vi "XVA-DSE7_defaut.vi"(8 "err in":errorcluster, 10 "tmax":dbl, 11 "Weibull (paramètres)":T1) -> (0 "err out":errorcluster, 2 "Graphe Weibull f et R":cluster{dbl[], dbl[]}[](graph) caption="Densité de Probabilité f et Fonction de Répartition F", 3 "X-VA (s)":T2)   [LabVIEW 2010, in "lv_04.lvlib"]
uses:
  lv_04.lvlib
  commandes/cX.ctl
  commandes/cSTA_varid.ctl
  commandes/c_TDMS_ch_variable.ctl
  commandes/c_TDMS_ch_donnees.ctl
  commandes/c0-var-n.ctl
  commandes/cSTA_num_do_cr.ctl
  commandes/c02-do-num.ctl
  commandes/c04-stat-num.ctl
  commandes/cSTA_txt_do_cr.ctl
  commandes/c02-do-txt.ctl
  commandes/c04-stat-txt.ctl
  commandes/cSTA_dist.ctl
  commandes/c03-dist-S.ctl
  commandes/c0-dist-xy.ctl
  commandes/c03-dist-T.ctl
  commandes/c03-dist-SPC.ctl
  lv_02/p_5E7_LW.ctl
  XVA-DSE7-dist.vi
  lv_02/lv_02.lvlib
panel:
  # "Loi Weibull"
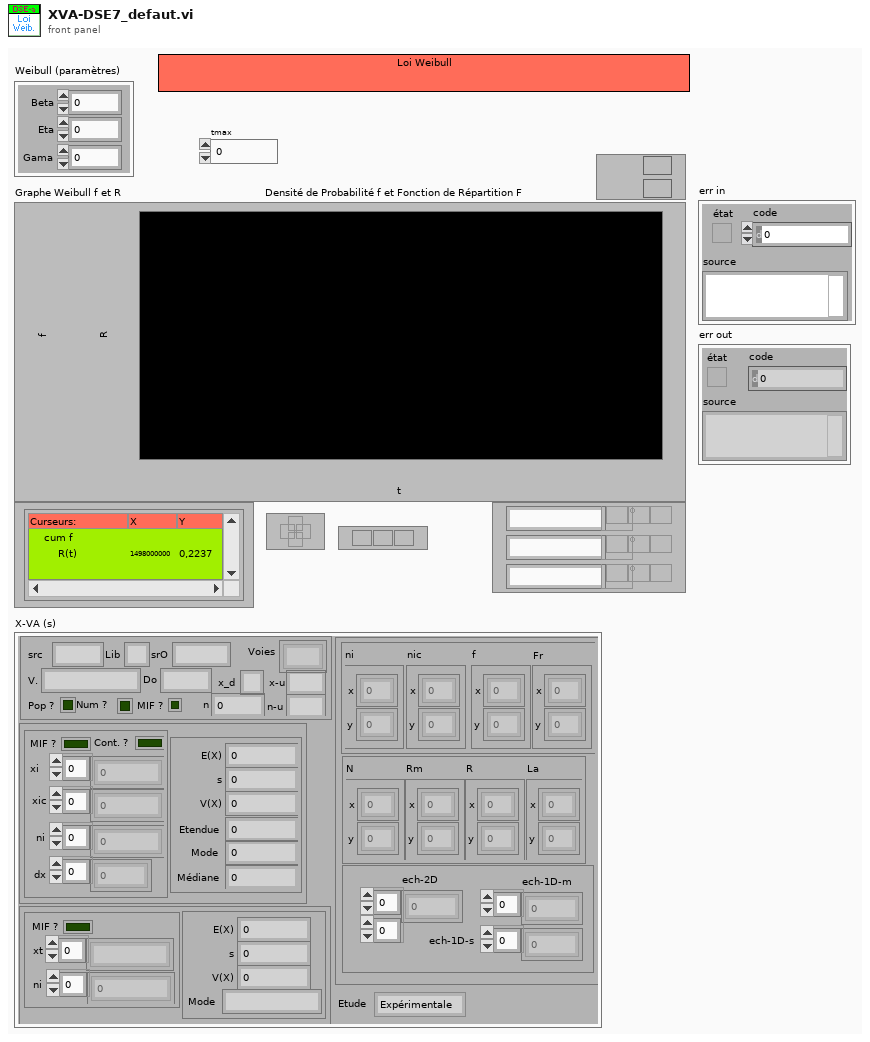
[diagram p1: front panel]
types:
  T1 = typedef "lv_02.lvlib/p_5E7_LW.ctl" = cluster{"Beta":dbl, "Eta":dbl, "Gama":dbl}
  T2 = typedef "lv_04.lvlib/cX.ctl" = cluster{"src":T3, "num":T7, "txt":T10, "dist":T13, "Etude":enum16{"Expérimentale", "Modèle"}}
  T3 = typedef "lv_04.lvlib/cSTA_varid.ctl" = cluster{"src":string, "Lib":string, "srO":string, "V.":T4, "Voies":string[], "Do":T5, "n":T6, "Num ?":bool, "Pop ?":bool, "x_d":string, "x-u":string, "n-u":string, "MIF ?":bool}
  T4 = typedef "lv_04.lvlib/c_TDMS_ch_variable.ctl" = string
  T5 = typedef "lv_04.lvlib/c_TDMS_ch_donnees.ctl" = string
  T6 = typedef "lv_04.lvlib/c0-var-n.ctl" = i32
  T7 = typedef "lv_04.lvlib/cSTA_num_do_cr.ctl" = cluster{"do":T8, "sta":T9}
  T8 = typedef "lv_04.lvlib/c02-do-num.ctl" = cluster{"MIF ?":bool, "Cont. ?":bool, "xi":dbl[], "xic":dbl[], "ni":u32[], "dx":dbl[]}
  T9 = typedef "lv_04.lvlib/c04-stat-num.ctl" = cluster{"E(X)":dbl, "s":dbl, "V(X) ":dbl, "Etendue":dbl, "Mode":dbl, "Médiane":dbl}
  T10 = typedef "lv_04.lvlib/cSTA_txt_do_cr.ctl" = cluster{"do":T11, "sta":T12}
  T11 = typedef "lv_04.lvlib/c02-do-txt.ctl" = cluster{"xt":string[], "ni":dbl[], "MIF ?":bool}
  T12 = typedef "lv_04.lvlib/c04-stat-txt.ctl" = cluster{"E(X)":dbl, "s":dbl, "V(X) ":dbl, "Mode":string}
  T13 = typedef "lv_04.lvlib/cSTA_dist.ctl" = cluster{"S":T14, "T":T16, "spc":T17}
  T14 = typedef "lv_04.lvlib/c03-dist-S.ctl" = cluster{"nic":T15, "f":T15, "Fr":T15, "ni":T15}
  T15 = typedef "lv_04.lvlib/c0-dist-xy.ctl" = cluster{"x":dbl[], "y":dbl[]}
  T16 = typedef "lv_04.lvlib/c03-dist-T.ctl" = cluster{"N":T15, "Rm":T15, "R":T15, "La":T15}
  T17 = typedef "lv_04.lvlib/c03-dist-SPC.ctl" = cluster{"ech-2D":dbl[][], "ech-1D-m":dbl[], "ech-1D-s":dbl[]}
  T18 = typedef "lv_01.lvlib/do_serie-c.ctl" = cluster{"X":dbl[], "par":cluster{"x_deb":dbl, "Pas":dbl, "Nb":dbl}}
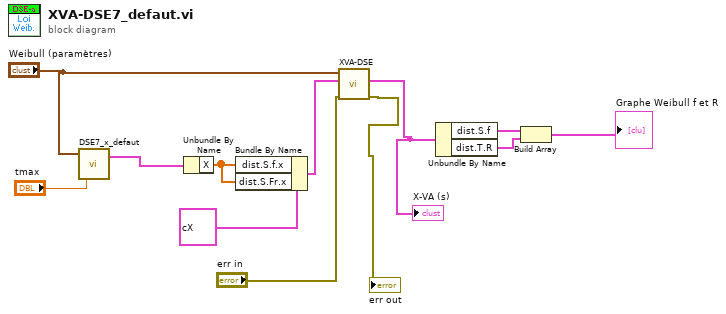
[diagram p0: block diagram]
diagram:
  n1 = call "DSE7_x_defaut.vi"("tmax"="tmax", "Weibull (paramètres)"="Weibull (paramètres)") -> ("sér. (s)"=w1:T18)  [unwired: 1 in]
  n2 = Unbundle By Name(w1) -> ("X"=w11:dbl[])
  n3 = Bundle By Name(cluster=T2 {"src"={"src"="", "Lib"="", "srO"="", "V."="", "Voies"=[], "Do"="", "n"=0, "Num ?"=FALSE, "Pop ?"=FALSE, "x_d"="", "x-u"="", "n-u"="", "MIF ?"=FALSE}, "num"={"do"={"MIF ?"=FALSE, "Cont. ?"=FALSE, "xi"=[], "xic"=[], "ni"=[], "dx"=[]}, "sta"={"E(X)"=0.0, "s"=0.0, "V(X) "=0.0, "Etendue"=0.0, "Mode"=0.0, "Médiane"=0.0}}, "txt"={"do"={"xt"=[], "ni"=[], "MIF ?"=FALSE}, "sta"={"E(X)"=0.0, "s"=0.0, "V(X) "=0.0, "Mode"=""}}, "dist"={"S"={"nic"={"x"=[], "y"=[]}, "f"={"x"=[], "y"=[]}, "Fr"={"x"=[], "y"=[]}, "ni"={"x"=[], "y"=[]}}, "T"={"N"={"x"=[], "y"=[]}, "Rm"={"x"=[], "y"=[]}, "R"={"x"=[], "y"=[]}, "La"={"x"=[], "y"=[]}}, "spc"={"ech-2D"=[], "ech-1D-m"=[], "ech-1D-s"=[]}}, "Etude"=enum."Expérimentale"} ("cXB (s)"), "dist.S.f.x"=w11, "dist.S.Fr.x"=w11) -> (w7:T2)
  n4 = call-poly "XVA-DSE.vi"("err in"="err in", "X-VA (e)"=w7, "p_LW"="Weibull (paramètres)") -> ("err out"=→"err out":errorcluster, "VA (s)"=w4:T2)  [unwired: 6 in, 1 out]
  "X-VA (s)" <- w4
  n5 = Unbundle By Name(w4) -> ("dist.S.f"=w10:T15, "dist.T.R"=w9:T15)
  n6 = Build Array(w10, w9) -> (→"Graphe Weibull f et R":T15[])
